vi "VISA open.vi"(8 "error in (no error)":errorcluster, 11 "Cobolt in":refnum<class "Cobolt.lvclass">) -> (0 "error out":errorcluster, 3 "Cobolt out":refnum<class "Cobolt.lvclass">)   [LabVIEW 2012, in "Cobolt.lvclass"]
uses:
  Cobolt.lvclass
  Cobolt.lvclass/Cobolt.ctl
  <vilib>/Instr/_visa.llb/VISA Configure Serial Port (Instr).vi
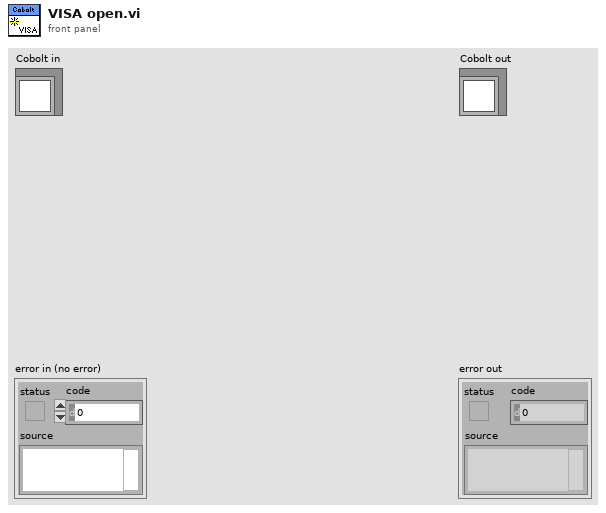
[diagram p1: front panel]
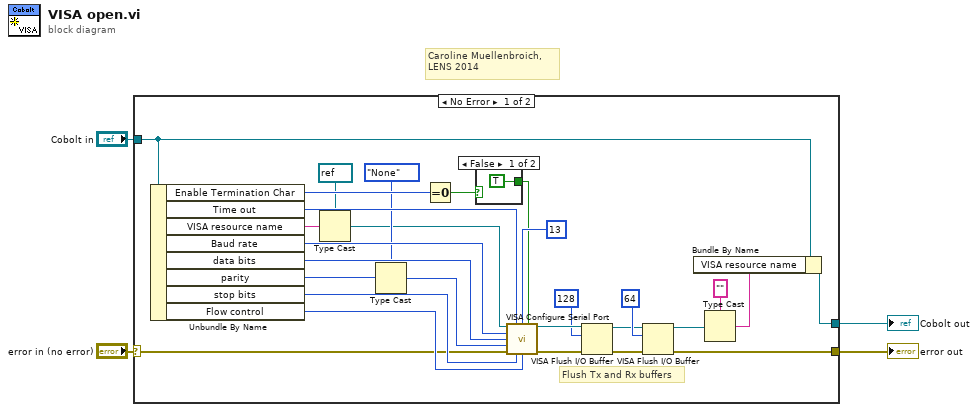
[diagram p0: block diagram]
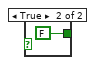
[diagram p2: hidden frame]
diagram:
  # "Caroline Muellenbroich, \nLENS 2014"
  n1 = case shown="No Error" "error in (no error)" {
    selector: "error in (no error)" -> [w8 w36]
    tunnel: [w7 w36] -> w3
    tunnel: [w5 w35] -> w1
    tunnel: "Cobolt in" -> [w6 w35]
    frame No Error {
      # "Flush Tx and Rx buffers"
      n2 = Unbundle By Name(w6) -> ("Enable Termination Char"=w21:u16, "Time out"=w24:u32, "VISA resource name"=w15:string, "Baud rate"=w23:u32, "data bits"=w16:u16, "parity"=w12:u16, "stop bits"=w14:u16, "Flow control"=w17:u16)
      n3 = Type Cast(type=refnum<visa-resource-name> refnum ("VISA resource name"), x=w15) -> (*(type *) &x=w10:refnum<visa-resource-name>)
      n4 = Type Cast(type=enum16{"None", "Odd", "Even", "Mark", "Space"}."None" ("parity (0:none)"), x=w12) -> (*(type *) &x=w13:enum16{"None", "Odd", "Even", "Mark", "Space"})
      n5 = Equal To 0?(x=w21) -> (x = 0?=w20:bool)
      n6 = case shown="False" w20 {
        tunnel: [TRUE FALSE] -> w22
        frame False {
        }
        frame True {
        }
      }
      n7 = call-poly "VISA Configure Serial Port"("VISA resource name"=w10, "timeout (10sec)"=w24, "termination char\n(0xA = '\\n' = LF)"=u8 13 ("termination char\n(0xA = '\\n' = LF)"), "Enable Termination\nChar (T)"=w22, "baud rate (9600)"=w23, "data bits (8)"=w16, "parity (0:none)"=w13, "error in (no error)"=w8, "stop bits (10: 1 bit)"=w14, "flow control (0:none)"=w17) -> ("VISA resource name out"=w31:refnum<visa-resource-name>, "error out"=w30:errorcluster)  [unwired: 4 in]
      n8 = VISA Flush I/O Buffer(VISA resource name=w31, mask (16)=u16 128, error in (no error)=w30) -> (VISA resource name out=w27:refnum<visa-resource-name>, error out=w26:errorcluster)
      n9 = VISA Flush I/O Buffer(VISA resource name=w27, mask (16)=u16 64, error in (no error)=w26) -> (VISA resource name out=w32:refnum<visa-resource-name>, error out=w7:errorcluster)
      n10 = Type Cast(type="" ("Configuration_cluster.VISA resource name"), x=w32) -> (*(type *) &x=w18:string)
      n11 = Bundle By Name(cluster=w6, "VISA resource name"=w18) -> (w5:refnum<class "Cobolt.lvclass">)
    }
    frame Error {
    }
  }
  "error out" <- w3
  "Cobolt out" <- w1
